vi "deinitialize.vi"(0 "HGF_DIMService":refnum<class "HGF_DIMService.lvclass">, 5 "error in (no error)":errorcluster) -> (19 "error out":errorcluster)   [LabVIEW 2012, in "HGF_DIM.lvlib" / "HGF_DIMService.lvclass"]
doc: "This is a dynamic dispatch VI. It can be overwritten by childclasses to release allocated recources."
uses:
  HGF_DIMService.lvclass
  HGF_BaseClasses/HGF_PVPublisher/HGF_PVPublisher.lvclass
  HGF_DIMService.lvclass/HGF_DIMService.ctl
  DimLVEvent/LVDimInterface/LVDimInterface.lvlib
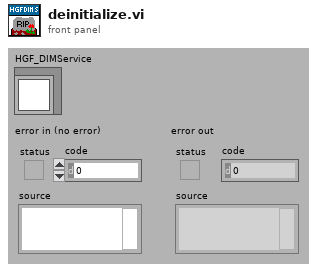
[diagram p1: front panel]
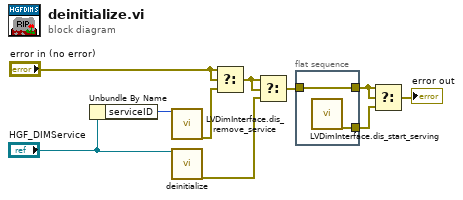
[diagram p0: block diagram]
diagram:
  n1 = Unbundle By Name("HGF_DIMService") -> ("serviceID"=w9:i32)
  n2 = call "LVDimInterface.dis_remove_service.vi"("my_serviceID"=w9) -> ("error out"=w7:errorcluster)  [unwired: 1 in, 17 out]
  n3 = call-parent "deinitialize.vi"("HGF_Factory"="HGF_DIMService") -> ("error out"=w5:errorcluster)  [unwired: 1 in, 17 out]
  n4 = Select(t="error in (no error)", s="error in (no error)", f=w7) -> (s? t:f=w6:errorcluster)
  n5 = Select(t=w6, s=w6, f=w5) -> (s? t:f=w4:errorcluster)
  n6 = flat-sequence {
    tunnel: w4 -> [w12]
    tunnel: [w12] -> w3
    tunnel: [w11] -> w2
    frame #0 {
      n7 = call "LVDimInterface.dis_start_serving.vi"() -> ("error out"=w11:errorcluster)  [unwired: 2 in, 17 out]
    }
  }
  n8 = Select(t=w3, s=w3, f=w2) -> (s? t:f=→"error out":errorcluster)
